vi "MM6Archiver.contents.vi"() -> ()   [LabVIEW 2014, in "MM6Archiver.lvlib"]
doc: "loads all VIs into memory required for building an application"
uses:
  MM6Archiver.lvlib
panel:
  out "error out":errorcluster
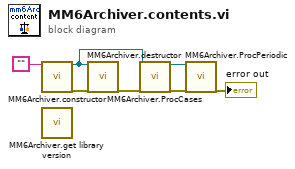
[diagram p0: block diagram]
diagram:
  n1 = call "MM6Archiver.constructor.vi"("name"="") -> ("i ref out"=w5:refnum<vi>, "error out"=w4:errorcluster)  [unwired: 16 in, 1 out]
  n2 = call "MM6Archiver.get library version.vi"() -> ()  [unwired: 1 in, 1 out]
  n3 = call "MM6Archiver.destructor.vi"("i ref in"=w5, "error in (no error)"=w4) -> ("error out"=w3:errorcluster)  [unwired: 17 in]
  n4 = call "MM6Archiver.ProcCases.vi"("i ref in"=w5, "error in (no error)"=w3) -> ("i ref out"=w6:refnum<vi>, "error out"=w2:errorcluster)  [unwired: 15 in, 1 out]
  n5 = call "MM6Archiver.ProcPeriodic.vi"("i ref in"=w6, "error in (no error)"=w2) -> ("error out"=→"error out":errorcluster)  [unwired: 15 in, 2 out]
